vi "Pause WS.vi"(4 "Secret ID (Default)":string, 5 "WS Name":string, 6 "Access ID (Default)":string, 8 "error in (no error)":errorcluster, 9 "Port":u16, 10 "Host":string, 11 "Scheme (HTTP)":T1) -> (0 "error out":errorcluster)   [LabVIEW 2020, in "WS Admin.lvlib"]
doc: "Pauses a Web Service so it stops responding to requests but stays deployed. For more description of the controls for this VI see the context help for <b>Do WS Action.vi</b>"
uses:
  WS Admin.lvlib
  Scheme.ctl
  Client Data.ctl
  HTTP Method.ctl
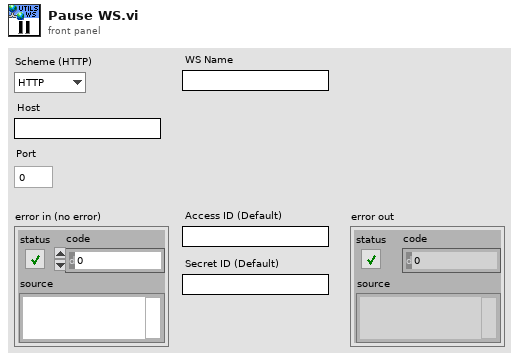
[diagram p1: front panel]
types:
  T1 = typedef "WS Admin.lvlib/Scheme.ctl" = enum16{"HTTP", "HTTPS"}
  T2 = typedef "WS Admin.lvlib/HTTP Method.ctl" = enum16{"GET", "POST", "PUT", "DELETE"}
  T3 = typedef "WS Admin.lvlib/Client Data.ctl" = cluster{"HTTP Method":T2, "URL Path":string, "Access ID":string, "Secret ID":string}
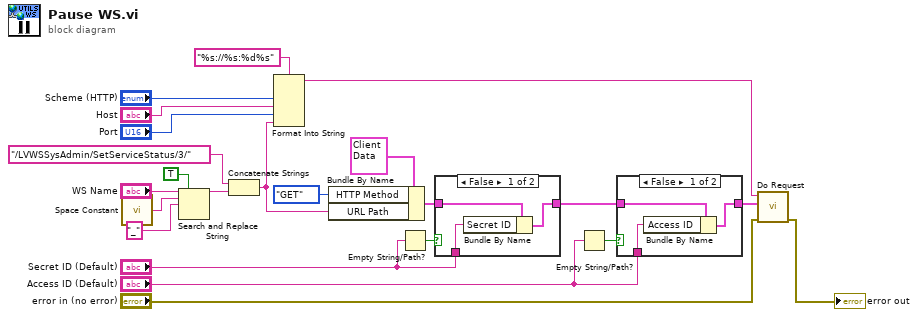
[diagram p0: block diagram]
diagram:
  n1 = call <vilib>:"Space Constant.vi"() -> ("String"=w22:string)
  n2 = Search and Replace String(replace all?=TRUE ("replace all? (F)"), input string="WS Name", search string=w22, replace string="_" ("replace string (\"\")")) -> (result string=w15:string)  [unwired: 4 in, 3 out]
  n3 = Concatenate Strings("/LVWSSysAdmin/SetServiceStatus/3/", w15) -> (w12:string)
  n4 = Format Into String(format string="%s://%s:%d%s", "Scheme (HTTP)", "Host", "Port", w12) -> (resulting string=w2:string)  [unwired: 2 in, 1 out]
  n5 = Bundle By Name(cluster=T3 {"HTTP Method"=enum."GET", "URL Path"="", "Access ID"="PqVr/ifkAQh+lVrdPIykXlFvg12GhhQFR8H9cUhphgg=", "Secret ID"="pTe9HRlQuMfJxAG6QCGq7UvoUpJzAzWGKy5SbZ+roSU="} ("Client Data"), "HTTP Method"=HTTP_Method."GET", "URL Path"=w12) -> (w9:T3)
  n6 = Empty String/Path?(string/path="Secret ID (Default)") -> (empty?=w10:bool)
  n7 = case shown="False" w10 {
    tunnel: w9 -> [w26 w27]
    tunnel: "Secret ID (Default)" -> [w25 _]
    tunnel: [w24 w27] -> w7
    frame False {
      n8 = Bundle By Name(cluster=w26, "Secret ID"=w25) -> (w24:T3)
    }
    frame True {
    }
  }
  n9 = Empty String/Path?(string/path="Access ID (Default)") -> (empty?=w6:bool)
  n10 = case shown="False" w6 {
    tunnel: w7 -> [w30 w31]
    tunnel: "Access ID (Default)" -> [w29 _]
    tunnel: [w28 w31] -> w4
    frame False {
      n11 = Bundle By Name(cluster=w30, "Access ID"=w29) -> (w28:T3)
    }
    frame True {
    }
  }
  n12 = call "Do Request.vi"("error in (no error)"="error in (no error)", "Client Data"=w4, "URL"=w2) -> ("error out"=→"error out":errorcluster)  [unwired: 7 in, 1 out]
